vi "Read Measurement (Normal).vi"(6 "Timeout (10000 ms)":i32=10000 min=1, 8 "error in (no error)":errorcluster, 9 "Number of Item (15)":i32=15 min=1 max=255, 10 "Measure Item (1: Plural)":i32(ring)=1 items=["One", "Plural"], 11 "VISA resource name":refnum<visa-resource-name>) -> (0 "error out":errorcluster, 1 "Measurement":dbl[](array[numeric]), 2 "Function":string[](array[string]), 3 "VISA resource name out":refnum<visa-resource-name>)   [LabVIEW 2023, in "Yokogawa WT300 Series.lvlib"]
doc: "Queries the numeric data."
uses:
  Yokogawa WT300 Series.lvlib
  Low Level/Fetch Measurement (Normal).vi
panel:
  # "ms"
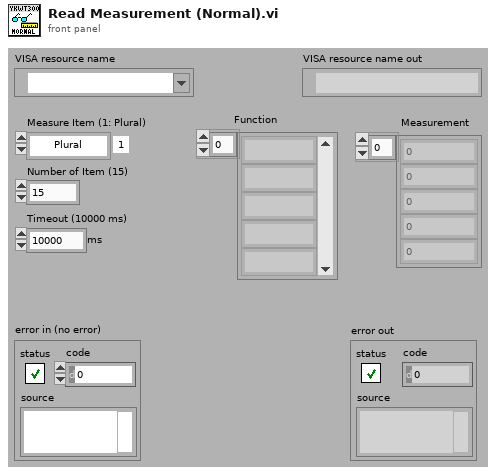
[diagram p1: front panel]
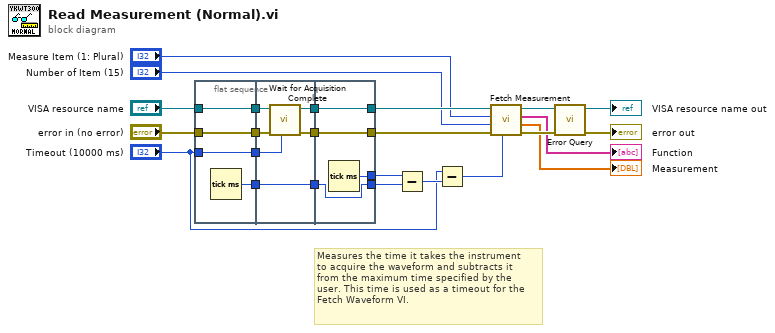
[diagram p0: block diagram]
diagram:
  # "Measures the time it takes the instrument \nto acquire the waveform and subtracts it \nfrom the maximum time specified by the \nuser. This time is used as a timeout for the \nFetch Waveform VI."
  n1 = flat-sequence {
    tunnel: "VISA resource name" -> [w27]
    tunnel: [w27] -> w7
    tunnel: "error in (no error)" -> [w26]
    tunnel: [w26] -> w6
    tunnel: [w28] -> w5
    tunnel: "Timeout (10000 ms)" -> [w25]
    tunnel: [w25] -> w4
    tunnel: w7 -> [w33]
    tunnel: [w31] -> w3
    tunnel: w6 -> [w32]
    tunnel: [w30] -> w2
    tunnel: w5 -> [w29]
    tunnel: [w29] -> w1
    tunnel: w4 -> [w34]
    tunnel: [w37] -> w23
    tunnel: w3 -> [w37]
    tunnel: [w36] -> w24
    tunnel: w2 -> [w36]
    tunnel: [w35] -> w21
    tunnel: w1 -> [w35]
    tunnel: [w38] -> w22
    frame #0 {
      n2 = Tick Count (ms)() -> (millisecond timer value=w28:u32)
    }
    frame #1 {
      n3 = call "Wait for Acquisition Complete.vi"("Timeout (10000 ms)"=w34, "error in (no error)"=w32, "VISA resource name"=w33) -> ("error out"=w30:errorcluster, "VISA resource name out"=w31:refnum<visa-resource-name>)  [unwired: 7 in]
    }
    frame #2 {
      n4 = Tick Count (ms)() -> (millisecond timer value=w38:u32)
    }
  }
  n5 = Subtract(x=w22, y=w21) -> (x-y=w19:u32)
  n6 = Subtract(x="Timeout (10000 ms)", y=w19) -> (x-y=w20:u32)
  n7 = call-poly "Fetch Measurement.vi"("Timeout (10000 ms)"=w20, "error in (no error)"=w24, "Number of Item (15)"="Number of Item (15)", "Measure Item (1: Plural)"="Measure Item (1: Plural)", "VISA resource name"=w23) -> ("error out"=w18:errorcluster, "Measurement"=→"Measurement":dbl[], "Function"=→"Function":string[], "VISA resource name out"=w17:refnum<visa-resource-name>)  [unwired: 3 in]
  n8 = call "Error Query.vi"("error in (no error)"=w18, "VISA resource name"=w17) -> ("error out"=→"error out":errorcluster, "VISA resource name out"=→"VISA resource name out":refnum<visa-resource-name>)  [unwired: 6 in, 2 out]
